vi "Sub Graph.vi"(10 "Length":i32=100, 11 "Graph":cluster{dbl[], dbl[]}) -> (3 "Sub Graph":cluster{dbl[], dbl[]})   [LabVIEW 2015]
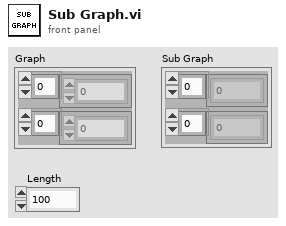
[diagram p1: front panel]
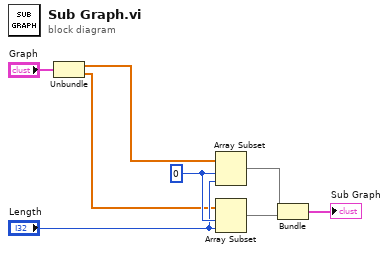
[diagram p0: block diagram]
diagram:
  w8 = 0 ("index")
  n1 = Unbundle("Graph") -> (w2:dbl[], w1:dbl[])
  n2 = Array Subset(array=w2, index=w8, length="Length") -> (w5:dbl[])
  n3 = Array Subset(array=w1, index=w8, length="Length") -> (w6:dbl[])
  n4 = Bundle(w5, w6) -> (→"Sub Graph":cluster{dbl[], dbl[]})  [unwired: 1 in]
